vi "Enable-Disable Data Acquisition.vi"(4 "error in (no error)":errorcluster, 6 "Data Acquisition Request (Disable)":bool, 7 "VISA resource name":refnum<visa-resource-name>) -> (0 "error out":errorcluster, 3 "VISA resource name out":refnum<visa-resource-name>)   [LabVIEW 2019, in "Newport ESP301.lvlib"]
doc: "This command is used to enable / disable the data acquisition request.\n<B>Note</B>: This command cannot be issued when:\n1. An axis is being homed (refer ASCII command, OR).\n2 .An axis is being moved to a travel limit (refer ASCII command, MT).\n3. An axis is being moved to an index (refer ASCII command, MZ)."
uses:
  Newport ESP301.lvlib
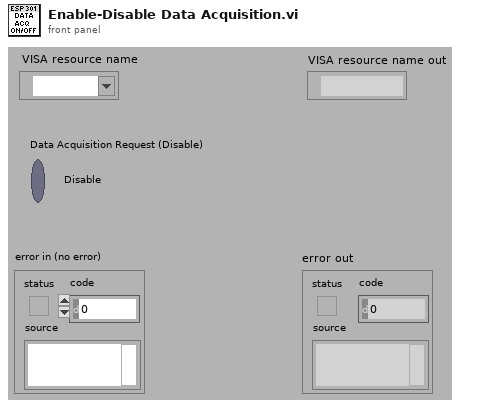
[diagram p1: front panel]
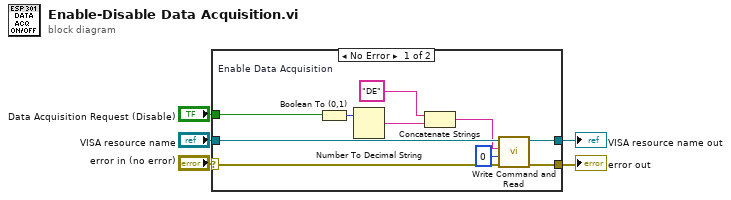
[diagram p0: block diagram]
diagram:
  n1 = case shown="No Error" "error in (no error)" {
    selector: "error in (no error)" -> [w12 w17]
    tunnel: [w14 w17] -> w5
    tunnel: "VISA resource name" -> [w15 w16]
    tunnel: [w13 w16] -> w4
    tunnel: "Data Acquisition Request (Disable)" -> [w8 _]
    frame No Error {
      w9 = "DE"  # Enable Data Acquisition
      n2 = Boolean To (0,1)(Boolean=w8) -> (0, 1=w10:i16)
      n3 = Number To Decimal String(number=w10) -> (decimal integer string=w11:string)  [unwired: 1 out]
      n4 = Concatenate Strings(w9, w11) -> (w7:string)
      n5 = call "Write Command and Read.vi"("error in (no error)"=w12, "Bytes to read (100)"=u32 0, "Command"=w7, "VISA resource name"=w15) -> ("error out"=w14:errorcluster, "VISA resource name out"=w13:refnum<visa-resource-name>)  [unwired: 1 in, 3 out]
    }
    frame Error {
    }
  }
  "error out" <- w5
  "VISA resource name out" <- w4
